vi "Read.vi"(8 "error in (no error)":errorcluster, 11 "HP3458aDMM in":refnum<class "HP3458aDMM.lvclass">) -> (0 "error out":errorcluster, 3 "HP3458aDMM out":refnum<class "HP3458aDMM.lvclass">)   [LabVIEW 2014, in "SamplerPlugins.lvlib" / "HP3458aDMM.lvclass"]
uses:
  HP3458aDMM.lvclass
  <instrlib>/Agilent 3458/Agilent 3458.lvlib
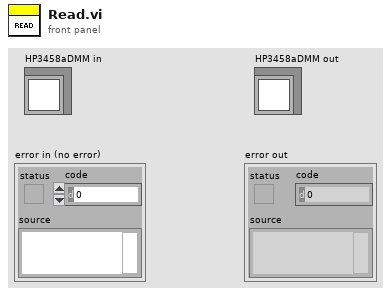
[diagram p1: front panel]
types:
  T1 = enum16{"ASCII", "Single Real", "Double Real", "Single Integer", "Double Integer"}
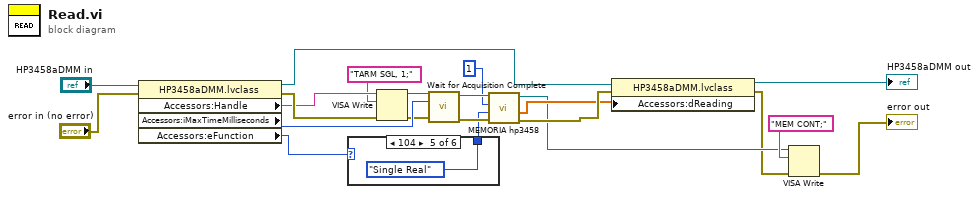
[diagram p0: block diagram]
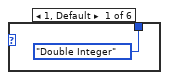
[diagram p2: hidden frame]
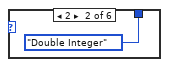
[diagram p3: hidden frame]
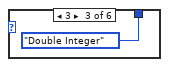
[diagram p4: hidden frame]
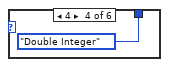
[diagram p5: hidden frame]
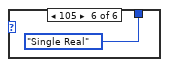
[diagram p6: hidden frame]
diagram:
  n1 = property class="HP3458aDMM.lvclass"(reference="HP3458aDMM in", error in="error in (no error)") -> (reference out=w18:refnum<class "HP3458aDMM.lvclass">, error out=w16:errorcluster, "Accessors:Handle"=w15:string, "Accessors:iMaxTimeMilliseconds"=w14:i32, "Accessors:eFunction"=w12:u16)
  n2 = case shown="104" w12 {
    tunnel: [T1."Double Integer" ("Output Format (0:ASCII)") T1."Double Integer" ("Output Format (0:ASCII)") T1."Double Integer" ("Output Format (0:ASCII)") T1."Double Integer" ("Output Format (0:ASCII)") T1."Single Real" ("Output Format (0:ASCII)") T1."Single Real" ("Output Format (0:ASCII)")] -> w1
    frame 1, Default {
    }
    frame 2 {
    }
    frame 3 {
    }
    frame 4 {
    }
    frame 104 {
    }
    frame 105 {
    }
  }
  n3 = VISA Write(VISA resource name=w15, write buffer="TARM SGL, 1;", error in (no error)=w16) -> (VISA resource name out=w6:refnum<visa-resource-name>, error out=w5:errorcluster)  [unwired: 1 out]
  n4 = call <instrlib>:"Wait for Acquisition Complete.vi"("error in (no error)"=w5, "Maximum Time (10000 ms)"=w14, "VISA resource name"=w6) -> ("error out"=w3:errorcluster, "VISA resource name out"=w4:refnum<visa-resource-name>)  [unwired: 7 in]
  n5 = call "MEMORIA hp3458.vi"("error in (no error)"=w3, "Output Format (0:ASCII)"=w1, "Número de muestras totales"=1, "VISA session"=w4) -> ("error out"=w17:errorcluster, "Muestras digitales"=w13:dbl[], "dup VISA session"=w10:refnum<visa-resource-name>)  [unwired: 4 in, 1 out]
  n6 = property class="HP3458aDMM.lvclass"(reference=w18, error in=w17, "Accessors:dReading"=w13) -> (reference out=→"HP3458aDMM out":refnum<class "HP3458aDMM.lvclass">, error out=w9:errorcluster)
  n7 = VISA Write(VISA resource name=w10, write buffer="MEM CONT;", error in (no error)=w9) -> (error out=→"error out":errorcluster)  [unwired: 2 out]
